vi "Get_SglVar_BulkMode_Value.vi"(8 "error in (no error)":errorcluster, 11 "muExpr in":refnum<class "mupExpr.lvclass">) -> (0 "error out":errorcluster, 2 "Value":dbl[](array[numeric]), 3 "muExpr out":refnum<class "mupExpr.lvclass">)   [LabVIEW 2015, in "mupExpr.lvclass"]
doc: "Return the expression's single variable's bulk mode values."
uses:
  mupExpr.lvclass
  mupExpr.lvclass/mupExpr.ctl
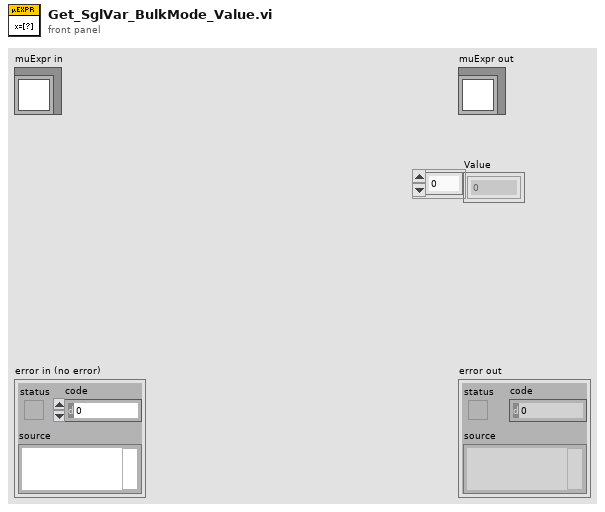
[diagram p1: front panel]
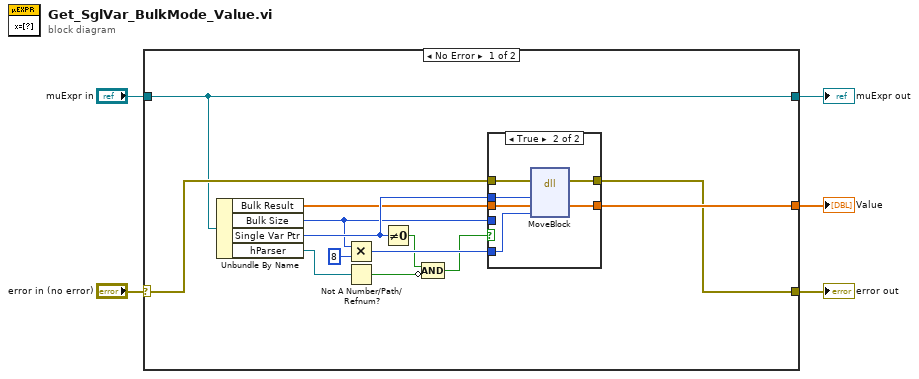
[diagram p0: block diagram]
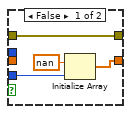
[diagram p2: hidden frame]
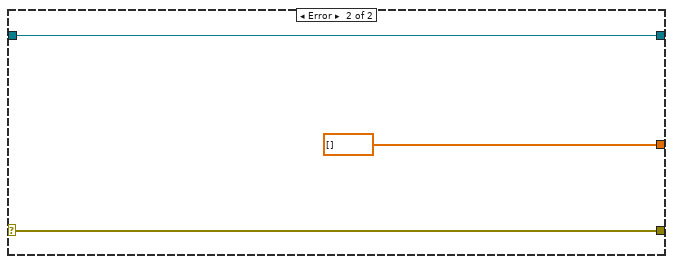
[diagram p3: hidden frame]
diagram:
  n1 = case shown="No Error" "error in (no error)" {
    selector: "error in (no error)" -> [w14 w31]
    tunnel: [w13 w31] -> w4
    tunnel: [w12 w30] -> w2
    tunnel: "muExpr in" -> [w12 w30]
    tunnel: [w18 dbl[] [] ("pd")] -> w1
    frame No Error {
      n2 = Unbundle By Name(w12) -> ("Bulk Result"=w11:dbl[], "Bulk Size"=w10:i32, "Single Var Ptr"=w17:u64, "hParser"=w9:refnum<data-value>)
      n3 = Multiply(x=w10, y=8 ("size")) -> (x*y=w15:i32)
      n4 = Not A Number/Path/Refnum?(number/path/refnum=w9) -> (NaN/Path/Refnum?=w7:bool)
      n5 = Not Equal To 0?(x=w17) -> (x != 0?=w8:bool)
      n6 = Compound Arithmetic op=AND(w8, invert w7) -> (w6:bool)
      n7 = case shown="True" w6 {
        tunnel: w11 -> [_ w28]
        tunnel: w14 -> [w22 w27]
        tunnel: [w22 w26] -> w13
        tunnel: w17 -> [_ w25]
        tunnel: [w19 w24] -> w18
        tunnel: w15 -> [_ w23]
        tunnel: w10 -> [w20 _]
        frame False {
          n8 = Initialize Array(nan ("pd"), w20) -> (w19:dbl[])
        }
        frame True {
          n9 = dll-call lib="LabVIEW" fn="MoveBlock"(error in=w27, "ps"=w25, "pd"=w28, "size"=w23) -> (error out=w26:errorcluster, "pd"=w24:dbl[])  [unwired: 5 in, 1 out]
        }
      }
    }
    frame Error {
    }
  }
  "error out" <- w4
  "muExpr out" <- w2
  "Value" <- w1
